vi "Do.vi"(8 "error in (no error)":cluster{"状态":bool, "代码":i32, "源":string} caption="错误输入（无错误）", 10 "操作者输入":refnum<class "Actor.lvclass">, 11 "goal_with_force_array_Msg消息":refnum<class "goal_with_force_array_Msg消息.lvclass">) -> (0 "error out":cluster{"状态":bool, "代码":i32, "源":string} caption="错误输出", 2 "操作者输出":refnum<class "Actor.lvclass">)   [LabVIEW 2014, in "GlobalPlannerPyPl.lvlib" / "goal_with_force_array_Msg消息.lvclass"]
doc: "本VI通过对操作者调用合适的方法，将消息发送给操作者。"
uses:
  <vilib>/ActorFramework/Actor/Actor.lvclass
  GlobalPlannerPyPlActor/GlobalPlannerPyPl.lvclass
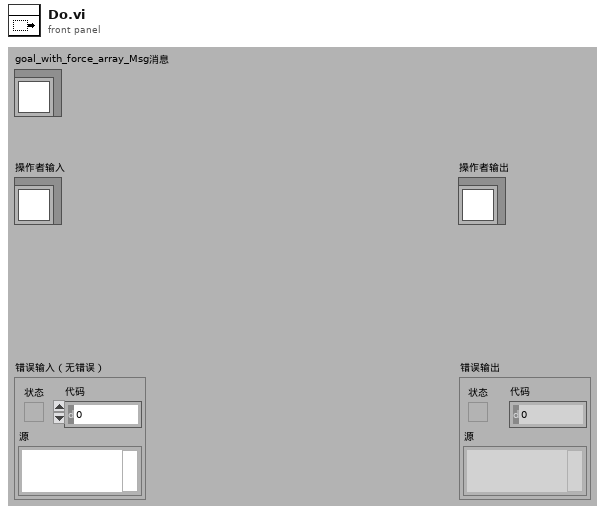
[diagram p1: front panel]
types:
  T1 = cluster{"pose_X":dbl, "pose_Y":dbl, "pose_z":dbl, "pose_rot":dbl, "force_bool":bool}[]
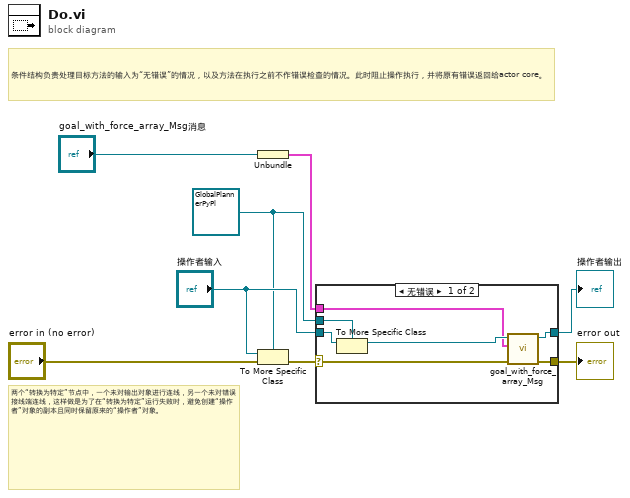
[diagram p0: block diagram]
diagram:
  w2 = refnum<class "GlobalPlannerPyPl.lvclass"> refnum ("Actor in")
  # "两个“转换为特定”节点中，一个未对输出对象进行连线，另一个未对错误接线端连线，这样做是为了在“转换为特定”运行失败时，避免创建“操作者”对象的副本且同时保留原来的“操作者”对象。"
  # "条件结构负责处理目标方法的输入为“无错误”的情况，以及方法在执行之前不作错误检查的情况。此时阻止操作执行，并将原有错误返回给actor core。"
  n1 = Unbundle("goal_with_force_array_Msg消息") -> (w1:T1)
  n2 = To More Specific Class(target class=w2, reference="操作者输入", error in="error in (no error)") -> (error out=w6:errorcluster)  [unwired: 1 out]
  n3 = case shown="无错误" w6 {
    selector: w6 -> [w13 w17]
    tunnel: [w15 w17] -> w5
    tunnel: [w14 w16] -> w4
    tunnel: "操作者输入" -> [w12 w16]
    tunnel: w2 -> [w11 _]
    tunnel: w1 -> [w9 _]
    frame No Error {
      n4 = To More Specific Class(target class=w11, reference=w12) -> (specific class reference=w10:refnum<class "GlobalPlannerPyPl.lvclass">)  [unwired: 1 in, 1 out]
      n5 = call-dynamic "goal_with_force_array_Msg.vi"("error in (no error)"=w13, "值(信号)"=w9, "GlobalPlannerPyPl输入"=w10) -> ("error out"=w15:errorcluster, "GlobalPlannerPyPl输出"=w14:refnum<class "GlobalPlannerPyPl.lvclass">)  [unwired: 7 in]
    }
    frame Error {
      # "如类型检查失败，则再次将原对象传出。"
    }
  }
  "error out" <- w5
  "操作者输出" <- w4
